vi "Display Song Library.vi"(8 "error in (no error)":errorcluster, 10 "Song Library":refnum<class "SongLibrary.lvclass">, 11 "SongBrowserActor in":refnum<class "SongBrowserActor.lvclass">) -> (0 "error out":errorcluster, 3 "SongBrowserActor out":refnum<class "SongBrowserActor.lvclass">)   [LabVIEW 2015, in "SongBrowserActor.lvlib" / "SongBrowserActor.lvclass"]
uses:
  SongBrowserActor.lvclass
  file/MusicElement/MusicElementLibrary/SongLibrary/SongLibrary.lvclass
  SongBrowserActor.lvclass/SongBrowserActor.ctl
  builds/xctls/Song Browser/Song Browser.lvlibp/app/xctls/Song Browser/Song Browser.xctl
  file/MusicElement/MusicElement.lvclass/MusicElement.ctl
  file/MusicElement/MusicElement.lvclass
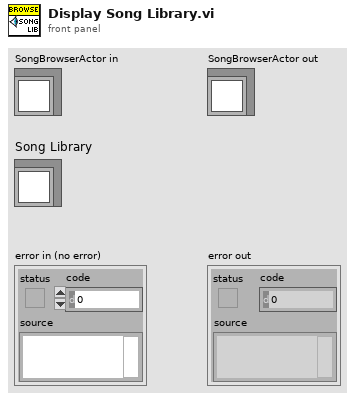
[diagram p1: front panel]
types:
  T1 = typedef "Song Browser Display.ctl" = cluster{"Song Name":string, "Artist":string, "Album":string, "Duration (s)":T2, "UID":string, "Enqueue":T3}
  T2 = typedef "Song.lvclass/Song Duration.ctl" = timestamp
  T3 = typedef "Enqueue Control.ctl" = bool
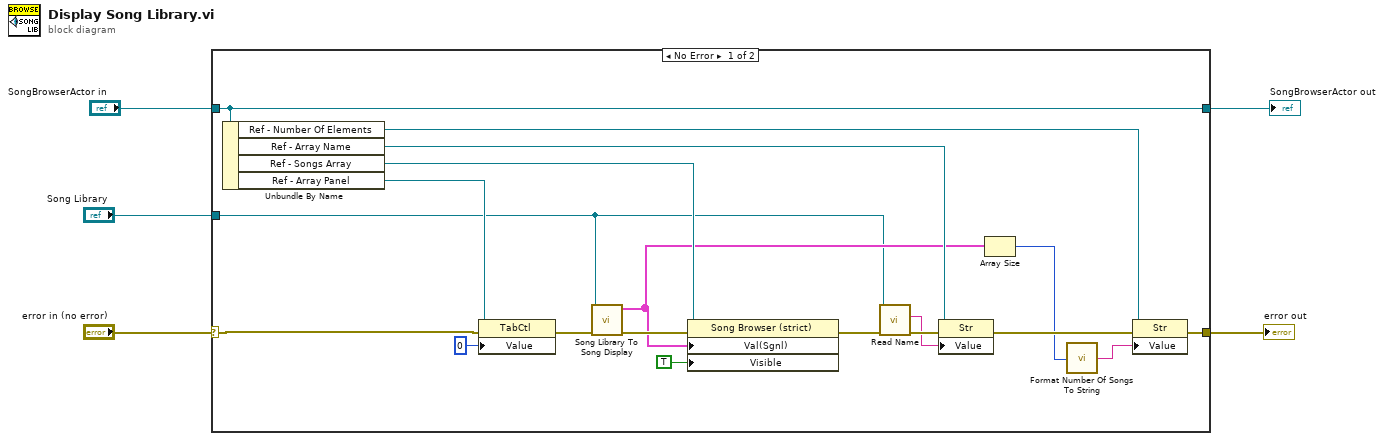
[diagram p0: block diagram]
diagram:
  n1 = case shown="No Error" "error in (no error)" {
    selector: "error in (no error)" -> [w10 w26]
    tunnel: [w17 w26] -> w4
    tunnel: [w24 w25] -> w2
    tunnel: "SongBrowserActor in" -> [w24 w25]
    tunnel: "Song Library" -> [w6 _]
    frame No Error {
      n2 = Unbundle By Name(w24) -> ("Ref - Number Of Elements"=w16:refnum<vi>, "Ref - Array Name"=w20:refnum<vi>, "Ref - Songs Array"=w22:refnum<vi>, "Ref - Array Panel"=w13:refnum<vi>)
      n3 = property class="TabCtl"(reference=w13, error in=w10, "Value"=0) -> (error out=w14:errorcluster)  [unwired: 1 out]
      n4 = call "Song Library To Song Display.vi"("error in (no error)"=w14, "Song Library"=w6) -> ("error out"=w23:errorcluster, "Songs"=w18:T1[])  [unwired: 8 in]
      n5 = property class="Song Browser (strict)"(reference=w22, error in=w23, "Val(Sgnl)"=w18, "Visible"=TRUE) -> (error out=w9:errorcluster)  [unwired: 1 out]
      n6 = call "Read Name.vi"("error in (no error)"=w9, "MusicElement in"=w6) -> ("error out"=w8:errorcluster, "Name"=w7:string)  [unwired: 7 in, 1 out]
      n7 = property class="Str"(reference=w20, error in=w8, "Value"=w7) -> (error out=w19:errorcluster)  [unwired: 1 out]
      n8 = Array Size(array=w18) -> (size(s)=w12:i32)
      n9 = call "Format Number Of Songs To String.vi"("Number Of Songs"=w12) -> ("Formatted"=w11:string)
      n10 = property class="Str"(reference=w16, error in=w19, "Value"=w11) -> (error out=w17:errorcluster)  [unwired: 1 out]
    }
    frame Error {
    }
  }
  "error out" <- w4
  "SongBrowserActor out" <- w2
